vi "Write Wiring Cluster.vi"(8 "error in (no error)":errorcluster, 10 "Wiring Configuration":T1, 11 "Control Experiment SM in":refnum<class "Control Experiment SM.lvclass">) -> (0 "error out":errorcluster, 3 "Control Experiment SM out":refnum<class "Control Experiment SM.lvclass">)   [LabVIEW 2016, in "Control Experiment SM.lvclass"]
uses:
  Control Experiment SM.lvclass
  Typedefs/Wiring Description--cluster.ctl
  Control Experiment SM.lvclass/Control Experiment SM.ctl
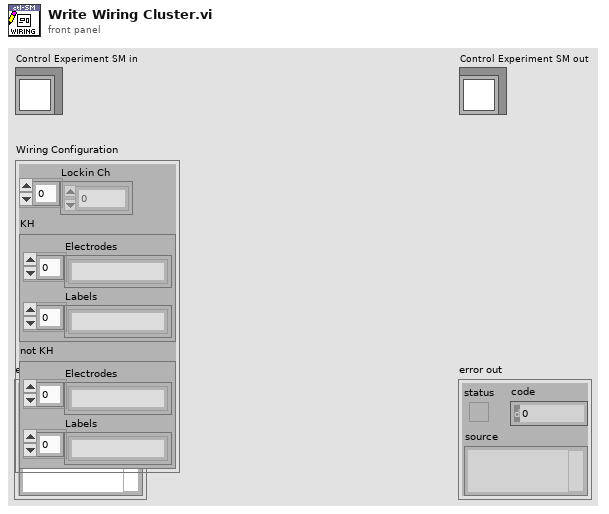
[diagram p1: front panel]
types:
  T1 = typedef "Control Experiment SM.lvclass/Wiring Description--cluster.ctl" = cluster{"Lockin Ch":i32[], "KH":cluster{"Electrodes":string[], "Labels":string[]}, "not KH":cluster{"Electrodes":string[], "Labels":string[]}}
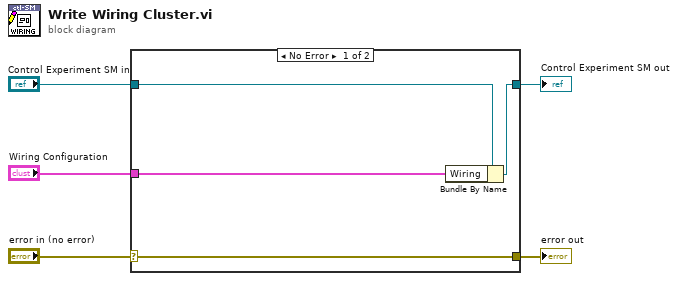
[diagram p0: block diagram]
diagram:
  n1 = case shown="No Error" "error in (no error)" {
    selector: "error in (no error)" -> [w9 w10]
    tunnel: [w9 w10] -> w4
    tunnel: [w7 w11] -> w2
    tunnel: "Control Experiment SM in" -> [w8 w11]
    tunnel: "Wiring Configuration" -> [w6 _]
    frame No Error {
      n2 = Bundle By Name(cluster=w8, "Wiring"=w6) -> (w7:refnum<class "Control Experiment SM.lvclass">)
    }
    frame Error {
    }
  }
  "error out" <- w4
  "Control Experiment SM out" <- w2
